vi "Dashboard Val Change.vi"(9 "OldVal":T1[](array[typedef]), 11 "NewVal":T1[](array[typedef])) -> ()   [LabVIEW 2015, in "SB SubVIs.lvlib"]
uses:
  SB SubVIs.lvlib
  Type Defs/Dashboard.ctl
  Globals.vi
  Globals (private).vi
  Type Defs/SB Type Defs.lvlib
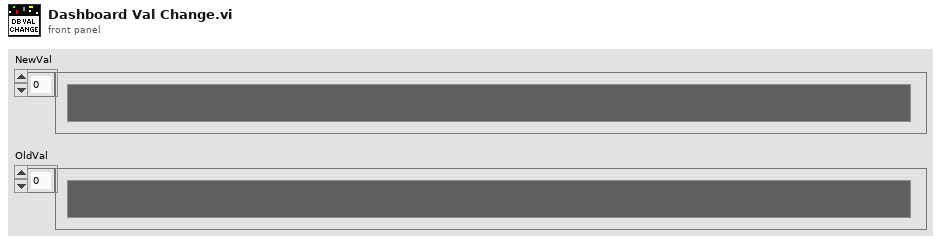
[diagram p1: front panel]
types:
  T1 = typedef "SB Type Defs.lvlib/Dashboard.ctl" = cluster{"Color":u32, "Player":i32, "Status":string, "Stats":string}
  T2 = typedef "SB Type Defs.lvlib/UI Refs.ctl" = cluster{"Battlefield":refnum<vi>, "Dashboard":refnum<vi>, "End Battle":refnum<vi>}
  T3 = cluster{"Color":u32, "Player Index":i32, "Status":string, "Stats":string}[]
  T4 = cluster{"Color":u32, "Player Index":i32, "Status":string, "Stats":string}
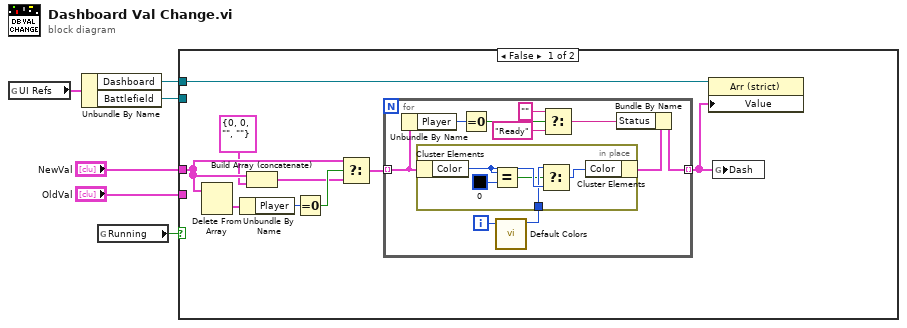
[diagram p0: block diagram]
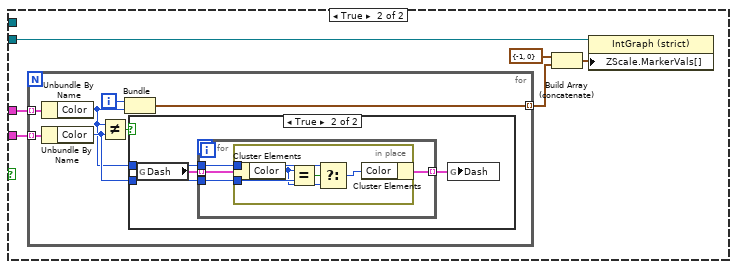
[diagram p2: hidden frame]
diagram:
  n1 = global read "Globals.vi" "UI Refs"() -> (w3:T2)
  n2 = Unbundle By Name(w3) -> ("Dashboard"=w2:refnum<vi>, "Battlefield"=w1:refnum<vi>)
  n3 = global read "Globals.vi" "Running"() -> (w6:bool)
  n4 = case shown="False" w6 {
    tunnel: w2 -> [w15 _]
    tunnel: "NewVal" -> [w10 w31]
    tunnel: "OldVal" -> [_ w32]
    tunnel: w1 -> [_ w33]
    frame False {
      n5 = Delete From Array(array=w10) -> (deleted portion=w14:T1)  [unwired: 2 in, 1 out]
      n6 = Unbundle By Name(w14) -> ("Player"=w13:i32)
      n7 = Build Array (concatenate)(w10, T1 {"Color"=0, "Player"=0, "Status"="", "Stats"=""} ("Dashboard")) -> (w9:T1[])
      n8 = Equal To 0?(x=w13) -> (x = 0?=w12:bool)
      n9 = Select(t=w10, s=w12, f=w9) -> (s? t:f=w11:T1[])
      n10 = for {
        tunnel: w11 -> [w21] mode=indexing
        tunnel: [w25] -> w7 mode=indexing
        i -> [w22]
        (unwired) T1 {"Color"=16777222, "Player"=0, "Status"="", "Stats"=""} ("Dashboard")
        n11 = Unbundle By Name(w21) -> ("Player"=w20:i32)
        n12 = Equal To 0?(x=w20) -> (x = 0?=w19:bool)
        n13 = call "Default Colors.vi"("Index"=w22) -> ("Color"=w24:u32)  [unwired: 10 in]
        n14 = in-place {
          in-place-border: w24 -> [w27]
          n15 = in-place-cluster #1(w21) -> ("Color"=w29:u32)
          n16 = Equal?(x=w29, y=u32 0) -> (x = y?=w26:bool)
          n17 = Select(t=w27, s=w26, f=w29) -> (s? t:f=w28:u32)
          n18 = in-place-cluster #1("Color"=w28) -> (w23:T1)
        }
        n19 = Select(t="", s=w19, f="Ready" ("Status")) -> (s? t:f=w16:string)
        n20 = Bundle By Name(cluster=w23, "Status"=w16) -> (w25:T1)
      }
      n21 = property class="Arr (strict)"(reference=w15, "Value"=w7) -> ()  [unwired: 1 in, 2 out]
      n22 = global write "Globals (private).vi" "Dash"(w7) -> ()
    }
    frame True {
      n23 = for {
        tunnel: w31 -> [w43] mode=indexing
        tunnel: [w41] -> w36 mode=indexing
        tunnel: w32 -> [w40] mode=indexing
        i -> [w42]
        n24 = Unbundle By Name(w43) -> ("Color"=w37:u32)
        n25 = Unbundle By Name(w40) -> ("Color"=w38:u32)
        n26 = Not Equal?(x=w37, y=w38) -> (x != y?=w39:bool)
        n27 = Bundle(w42, "Color"=w37) -> (w41:cluster{i32, "Color":u32})  [unwired: 1 in]
        n28 = case shown="True" w39 {
          tunnel: w38 -> [_ w45]
          tunnel: w37 -> [_ w44]
          frame False {
          }
          frame True {
            n29 = global read "Globals (private).vi" "Dash"() -> (w47:T3)
            n30 = for {
              tunnel: w47 -> [w51] mode=indexing
              tunnel: [w50] -> w46 mode=indexing
              tunnel: w45 -> [w49]
              tunnel: w44 -> [w48]
              n31 = in-place {
                in-place-border: w49 -> [w56]
                in-place-border: w48 -> [w54]
                n32 = in-place-cluster #2(w51) -> ("Color"=w53:u32)
                n33 = Equal?(x=w53, y=w56) -> (x = y?=w55:bool)
                n34 = Select(t=w54, s=w55, f=w53) -> (s? t:f=w52:u32)
                n35 = in-place-cluster #2("Color"=w52) -> (w50:T4)
              }
            }
            n36 = global write "Globals (private).vi" "Dash"(w46) -> ()
          }
        }
      }
      n37 = Build Array (concatenate)(cluster{i32, u32} {-1, 0} ("output cluster"), w36) -> (w34:cluster{i32, "Color":u32}[])
      n38 = property class="IntGraph (strict)"(reference=w33, "ZScale.MarkerVals[]"=w34) -> ()  [unwired: 1 in, 2 out]
    }
  }
